vi "Finish.vi"   [LabVIEW 2015]
doc: "This VI is called just before exiting. It is expected to close I/O refnum, save collected data, etc."
uses:
  <vilib>/Rock Robotics/WPI/Utilities/WPI_GetSetVariantRefNum.vi
  NavX/navX Library v2/navX Library v2.lvlib
types:
  T1 = typedef "navX Library v2.lvlib/Z900_navX_DeviceTypeDef.ctl" = cluster{"Interface":cluster{"Protocol":T2, "Update Rate (4Hz-60Hz)":u8, "navX Open TypeDef":variant}, "Notify Packet":refnum<notifier>, "Loop VI Refnum":refnum<vi>, "Ready to Close Occurrence Refnum":refnum<k4>}
  T2 = typedef "navX Library v2.lvlib/Z900_navX_ProtocolTypeDef.ctl" = enum16{"SERIAL", "I2C", "SPI"}
  T3 = typedef "WPI_SolenoidDevRef.ctl" = cluster{"DevStatus":errorcluster, "Pneumatics Control Module":u8, "Forward Solenoid Channel":T4, "Reverse Solenoid Channel":T4}
  T4 = typedef "WPI_SolenoidChannel.ctl" = enum8{"Solenoid 0", "Solenoid 1", "Solenoid 2", "Solenoid 3", "Solenoid 4", "Solenoid 5", "Solenoid 6", "Solenoid 7", "Invalid"}
  T5 = typedef "WPI_GyroDevRef.ctl" = cluster{"DevStatus":errorcluster, "Analog Channel":T6, "Offset":dbl, "Gain (VoltsPerDegree/Second)":dbl, "Gyro Type":enum16{"Analog", "XRS450"}, "Handle":i32, "SPI Bus":T7, "Device Found":bool, "Sample Rate":dbl, "Calibrate On Open":bool}
  T6 = typedef "FPGA_AIChannel.ctl" = enum8{"AI 0", "AI 1", "AI 2", "AI 3", "AI MXP 0", "AI MXP 1", "AI MXP 2", "AI MXP 3", "Invalid"}
  T7 = typedef "spi_bus.ctl" = enum16{"SPI On-Board, CS0", "SPI On-Board, CS1", "SPI On-Board, CS2", "SPI On-Board, CS3", "SPI MXP", "Invalid"}
  T8 = typedef "WPI_MotorControlDeviceRef.ctl" = cluster{"DeviceStatus":errorcluster, "Type":T9, "PWM":cluster{"PWM Channel":T10, "DeadBand":T11}, "CAN":cluster{"Device Number":u8, "Control Mode":T12, "Semaphore":T13, "Max Vout":dbl, "TalonSRX Control Mode":T14}, "Invert":bool}
  T9 = typedef "WPI_MotorControlType.ctl" = enum16{"PWM", "CAN", "CANTalonSRX"}
  T10 = typedef "FPGA_DIOPWMChannel.ctl" = enum8{"PWM 0", "PWM 1", "PWM 2", "PWM 3", "PWM 4", "PWM 5", "PWM 6", "PWM 7", "PWM 8", "PWM 9", "PWM MXP 0", "PWM MXP 1", "PWM MXP 2", "PWM MXP 3", "PWM MXP 4", "PWM MXP 5", "PWM MXP 6", "PWM MXP 7", "PWM MXP 8", "PWM MXP 9", "Invalid"}
  T11 = typedef "WPI_PWMDeadband.ctl" = cluster{"Name":string, "maxPositivePwm":i32, "minPositivePwm":i32, "centerPwm":i32, "maxNegativePwm":i32, "minNegativePwm":i32, "angularRange":u16}
  T12 = typedef "WPI_CANJaguar_ControlMode.ctl" = enum8{"Percent VBus", "Current", "Speed", "Position", "Voltage"}
  T13 = typedef "Semaphore RefNum" = refnum<k1>
  T14 = typedef "WPI_CANTalonSRX_APIControlMode.ctl" = enum8{"Percent VBus", "Speed", "Position", "Slave", "Unchanged / Invalid", "Voltage Compensation", "Current", "Motion Profile"}
  T15 = typedef "WPI_EncoderDevRef.ctl" = cluster{"DevStatus":errorcluster, "EncoderIndex":T16, "CounterIndex":T17, "DistancePerCount":dbl, "Decoding Type":T18}
  T16 = typedef "FPGA_EncoderIdx.ctl" = enum8{"Enc 0", "Enc 1", "Enc 2", "Enc 3", "Enc 4", "Enc 5", "Enc 6", "Enc 7", "Invalid"}
  T17 = typedef "FPGA_CounterCtrSystemIndex.ctl" = enum8{"Ctr 0", "Ctr 1", "Ctr 2", "Ctr 3", "Ctr 4", "Ctr 5", "Ctr 6", "Ctr 7", "Invalid"}
  T18 = typedef "WPI_EncoderType.ctl" = enum16{"1x", "2x", "4x"}
  T19 = typedef "WPI_DigitalInputDevRef.ctl" = cluster{"DevStatus":errorcluster, "DIO Channel":T20}
  T20 = typedef "FPGA_DIOChannel.ctl" = enum8{"DIO 0", "DIO 1", "DIO 2", "DIO 3", "DIO 4", "DIO 5", "DIO 6", "DIO 7", "DIO 8", "DIO 9", "DIO MXP 0", "DIO MXP 1", "DIO MXP 2", "DIO MXP 3", "DIO MXP 4", "DIO MXP 5", "DIO MXP 6", "DIO MXP 7", "DIO MXP 8", "DIO MXP 9", "DIO MXP 10", "DIO MXP 11", "DIO MXP 12", "DIO MXP 13", "DIO MXP 14", "DIO MXP 15", "Invalid"}
  T21 = typedef "WPI_JoystickDevRef.ctl" = cluster{"Device":T22}
  T22 = typedef "WPI_JoystickDeviceEnum.ctl" = enum16{"USB 0", "USB 1", "USB 2", "USB 3", "USB 4", "USB 5"}
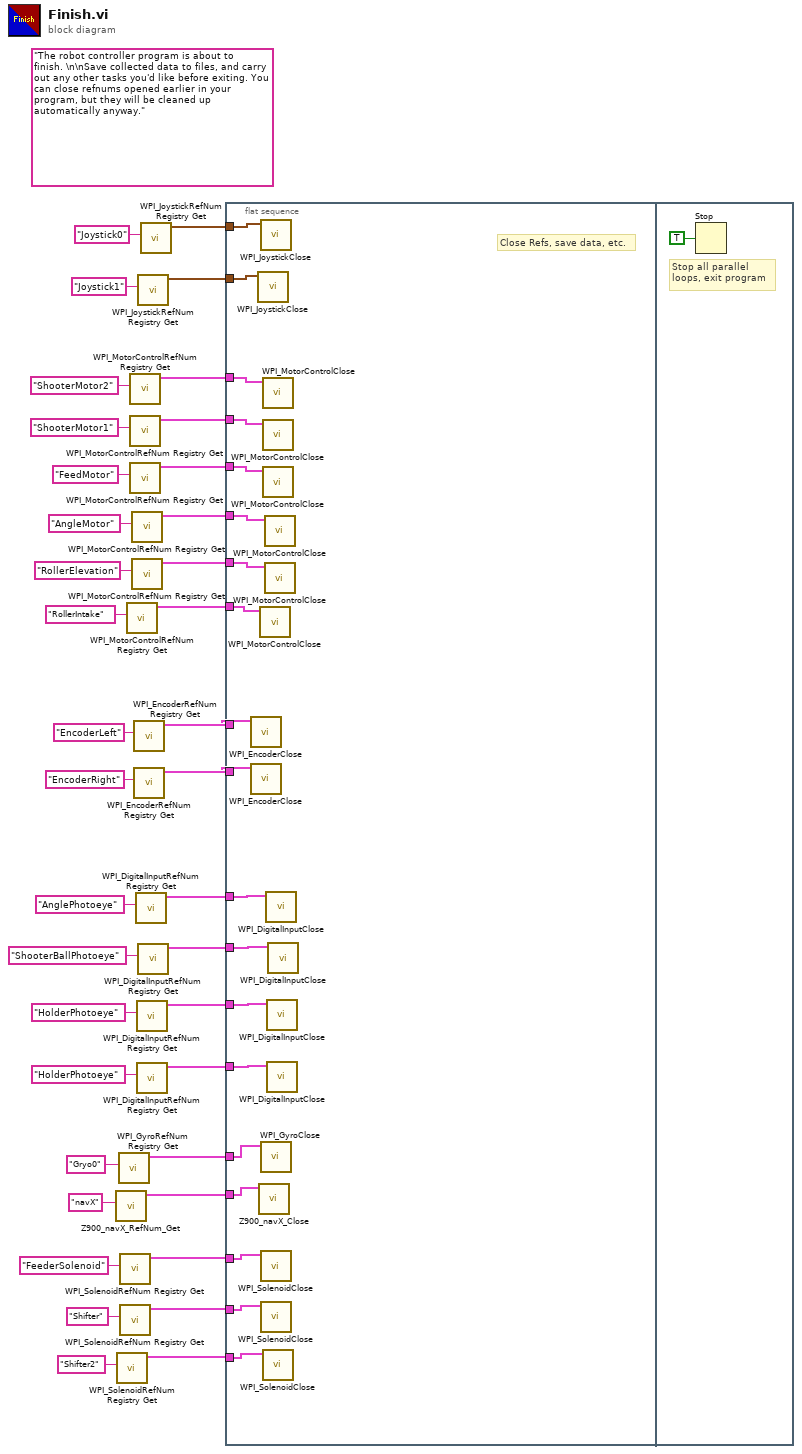
[diagram p0: block diagram]
diagram:
  (unwired) "The robot controller program is about to finish. \n\nSave collected data to files, and carry out any other tasks you'd like before exiting. You can close refnums opened earlier in your program, but they will be cleaned up automatically anyway."
  n1 = call "Z900_navX_RefNum_Get.vi"("refnum name"="navX") -> ("navX Device"=w1:T1)  [unwired: 9 in, 1 out]
  n2 = call <vilib>:"WPI_SolenoidRefNum Registry Get.vi"("refnum name"="Shifter2") -> ("SolenoidDevRef"=w3:T3)  [unwired: 9 in, 1 out]
  n3 = call <vilib>:"WPI_GyroRefNum Registry Get.vi"("refnum name"="Gryo0") -> ("GyroDevRef"=w10:T5)  [unwired: 9 in, 1 out]
  n4 = call <vilib>:"WPI_SolenoidRefNum Registry Get.vi"("refnum name"="FeederSolenoid") -> ("SolenoidDevRef"=w5:T3)  [unwired: 9 in, 1 out]
  n5 = call <vilib>:"WPI_SolenoidRefNum Registry Get.vi"("refnum name"="Shifter") -> ("SolenoidDevRef"=w4:T3)  [unwired: 9 in, 1 out]
  n6 = call <vilib>:"WPI_MotorControlRefNum Registry Get.vi"("refnum name"="RollerIntake") -> ("MotorControlDevRef"=w21:T8)  [unwired: 9 in, 1 out]
  n7 = call <vilib>:"WPI_MotorControlRefNum Registry Get.vi"("refnum name"="ShooterMotor2") -> ("MotorControlDevRef"=w30:T8)  [unwired: 9 in, 1 out]
  n8 = call <vilib>:"WPI_MotorControlRefNum Registry Get.vi"("refnum name"="ShooterMotor1") -> ("MotorControlDevRef"=w31:T8)  [unwired: 9 in, 1 out]
  n9 = call <vilib>:"WPI_MotorControlRefNum Registry Get.vi"("refnum name"="FeedMotor") -> ("MotorControlDevRef"=w32:T8)  [unwired: 9 in, 1 out]
  n10 = call <vilib>:"WPI_MotorControlRefNum Registry Get.vi"("refnum name"="AngleMotor") -> ("MotorControlDevRef"=w26:T8)  [unwired: 9 in, 1 out]
  n11 = call <vilib>:"WPI_MotorControlRefNum Registry Get.vi"("refnum name"="RollerElevation") -> ("MotorControlDevRef"=w25:T8)  [unwired: 9 in, 1 out]
  n12 = call <vilib>:"WPI_EncoderRefNum Registry Get.vi"("refnum name"="EncoderLeft") -> ("EncoderDevRef"=w14:T15)  [unwired: 9 in, 1 out]
  n13 = call <vilib>:"WPI_EncoderRefNum Registry Get.vi"("refnum name"="EncoderRight") -> ("EncoderDevRef"=w11:T15)  [unwired: 9 in, 1 out]
  n14 = call <vilib>:"WPI_DigitalInputRefNum Registry Get.vi"("refnum name"="AnglePhotoeye") -> ("DigitalInputDevRef"=w29:T19)  [unwired: 9 in, 1 out]
  n15 = call <vilib>:"WPI_DigitalInputRefNum Registry Get.vi"("refnum name"="HolderPhotoeye") -> ("DigitalInputDevRef"=w17:T19)  [unwired: 9 in, 1 out]
  n16 = call <vilib>:"WPI_DigitalInputRefNum Registry Get.vi"("refnum name"="HolderPhotoeye") -> ("DigitalInputDevRef"=w16:T19)  [unwired: 9 in, 1 out]
  n17 = call <vilib>:"WPI_JoystickRefNum Registry Get.vi"("refnum name"="Joystick1") -> ("JoystickDevRef"=w28:T21)  [unwired: 1 in, 9 out]
  n18 = call <vilib>:"WPI_DigitalInputRefNum Registry Get.vi"("refnum name"="ShooterBallPhotoeye") -> ("DigitalInputDevRef"=w20:T19)  [unwired: 9 in, 1 out]
  n19 = call <vilib>:"WPI_JoystickRefNum Registry Get.vi"("refnum name"="Joystick0") -> ("JoystickDevRef"=w37:T21)  [unwired: 1 in, 9 out]
  n20 = flat-sequence {
    tunnel: w37 -> [w57]
    tunnel: w32 -> [w56]
    tunnel: w31 -> [w55]
    tunnel: w30 -> [w54]
    tunnel: w29 -> [w53]
    tunnel: w28 -> [w52]
    tunnel: w25 -> [w50]
    tunnel: w26 -> [w51]
    tunnel: w21 -> [w49]
    tunnel: w20 -> [w48]
    tunnel: w17 -> [w47]
    tunnel: w16 -> [w46]
    tunnel: w14 -> [w45]
    tunnel: w11 -> [w44]
    tunnel: w10 -> [w43]
    tunnel: w5 -> [w42]
    tunnel: w4 -> [w41]
    tunnel: w3 -> [w40]
    tunnel: w1 -> [w39]
    frame #0 {
      # "Close Refs, save data, etc."
      n21 = call <vilib>:"WPI_EncoderClose.vi"("EncoderDevRef"=w45) -> ()  [unwired: 10 in, 1 out]
      n22 = call <vilib>:"WPI_EncoderClose.vi"("EncoderDevRef"=w44) -> ()  [unwired: 10 in, 1 out]
      n23 = call <vilib>:"WPI_JoystickClose.vi"("JoystickDevRef"=w52) -> ()  [unwired: 11 out]
      n24 = call "Z900_navX_Close.vi"("navX Device"=w39) -> ()  [unwired: 10 in, 1 out]
      n25 = call <vilib>:"WPI_MotorControlClose.vi"("MotorControlDevRef"=w49) -> ()  [unwired: 10 in, 1 out]
      n26 = call <vilib>:"WPI_JoystickClose.vi"("JoystickDevRef"=w57) -> ()  [unwired: 11 out]
      n27 = call <vilib>:"WPI_GyroClose.vi"("GyroDevRef"=w43) -> ()  [unwired: 10 in, 1 out]
      n28 = call <vilib>:"WPI_SolenoidClose.vi"("SolenoidDevRef"=w42) -> ()  [unwired: 10 in, 1 out]
      n29 = call <vilib>:"WPI_SolenoidClose.vi"("SolenoidDevRef"=w41) -> ()  [unwired: 10 in, 1 out]
      n30 = call <vilib>:"WPI_MotorControlClose.vi"("MotorControlDevRef"=w54) -> ()  [unwired: 10 in, 1 out]
      n31 = call <vilib>:"WPI_MotorControlClose.vi"("MotorControlDevRef"=w55) -> ()  [unwired: 10 in, 1 out]
      n32 = call <vilib>:"WPI_MotorControlClose.vi"("MotorControlDevRef"=w56) -> ()  [unwired: 10 in, 1 out]
      n33 = call <vilib>:"WPI_SolenoidClose.vi"("SolenoidDevRef"=w40) -> ()  [unwired: 10 in, 1 out]
      n34 = call <vilib>:"WPI_MotorControlClose.vi"("MotorControlDevRef"=w51) -> ()  [unwired: 10 in, 1 out]
      n35 = call <vilib>:"WPI_MotorControlClose.vi"("MotorControlDevRef"=w50) -> ()  [unwired: 10 in, 1 out]
      n36 = call <vilib>:"WPI_DigitalInputClose.vi"("DigitalInputDevRef"=w53) -> ()  [unwired: 10 in, 1 out]
      n37 = call <vilib>:"WPI_DigitalInputClose.vi"("DigitalInputDevRef"=w47) -> ()  [unwired: 10 in, 1 out]
      n38 = call <vilib>:"WPI_DigitalInputClose.vi"("DigitalInputDevRef"=w46) -> ()  [unwired: 10 in, 1 out]
      n39 = call <vilib>:"WPI_DigitalInputClose.vi"("DigitalInputDevRef"=w48) -> ()  [unwired: 10 in, 1 out]
    }
    frame #1 {
      # "Stop all parallel\nloops, exit program"
      n40 = Stop(stop? (T)=TRUE ("Quit")) -> ()
    }
  }
